vi "uA_daq_calculate_All_values_from Sub_chart.vi"(6 "Cursor.Cursor X 2":dbl, 9 "Cursor.Cursor X":dbl, 10 "Value":waveform(sgl), 11 "Sample rate":dbl) -> (0 "Sample":i32, 1 "Max value":dbl, 2 "Average":dbl, 3 "Delta(s)":sgl, 4 "Min value":dbl)   [LabVIEW 2017]
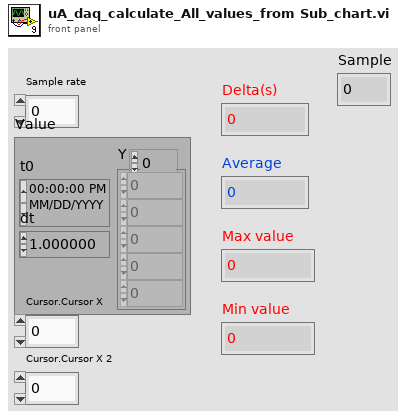
[diagram p1: front panel]
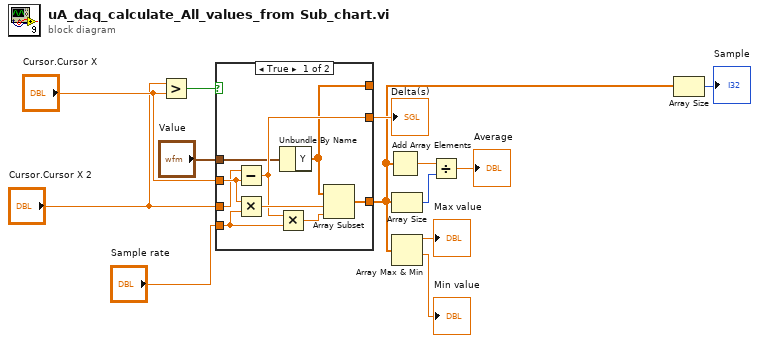
[diagram p0: block diagram]
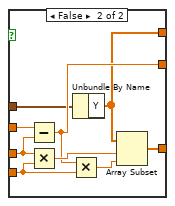
[diagram p2: hidden frame]
diagram:
  n1 = Greater?(x="Cursor.Cursor X 2", y="Cursor.Cursor X") -> (0:w3:bool)
  n2 = case shown="True" w3 {
    tunnel: "Value" -> [w16 w25]
    tunnel: "Cursor.Cursor X 2" -> [w18 w28]
    tunnel: "Cursor.Cursor X" -> [w19 w27]
    tunnel: [w20 w29] -> w2
    tunnel: [w17 w26] -> w9
    tunnel: "Sample rate" -> [w15 w24]
    tunnel: [w14 w23] -> _
    frame True {
      n3 = Subtract(x=w18, y=w19) -> (x-y=w17:dbl)
      n4 = Multiply(x=w19, y=w15) -> (x*y=w22:dbl)
      n5 = Multiply(x=w17, y=w15) -> (x*y=w21:dbl)
      n6 = Unbundle By Name(w16) -> ("Y"=w14:sgl[])
      n7 = Array Subset(array=w14, index=w22, length=w21) -> (w20:sgl[])
    }
    frame False {
      n8 = Subtract(x=w27, y=w28) -> (x-y=w26:dbl)
      n9 = Multiply(x=w28, y=w24) -> (x*y=w31:dbl)
      n10 = Multiply(x=w26, y=w24) -> (x*y=w30:dbl)
      n11 = Unbundle By Name(w25) -> ("Y"=w23:sgl[])
      n12 = Array Subset(array=w23, index=w31, length=w30) -> (w29:sgl[])
    }
  }
  "Delta(s)" <- w9
  n13 = Add Array Elements(numeric array=w2) -> (sum=w6:sgl)
  n14 = Array Size(array=w2) -> (size(s)=w7:i32)
  n15 = Array Max & Min(array=w2) -> (max value=→"Max value":sgl, min value=→"Min value":sgl)  [unwired: 2 out]
  n16 = Divide(x=w6, y=w7) -> (x/y=→"Average":sgl)
  n17 = Array Size(array=w2) -> (size(s)=→"Sample":i32)
